vi "Acquisition Done.vi"(8 "error in (no error)":errorcluster, 11 "Picam in":refnum<class "Picam.lvclass">) -> (0 "error out":errorcluster, 2 "Done":bool, 3 "Picam out":refnum<class "Picam.lvclass">)   [LabVIEW 2019, in "Picam.lvclass"]
uses:
  Picam.lvclass
  Picam.lvclass/Picam.ctl
  picam32_LabView_SDK/PICam_lib/PICam.lvlib
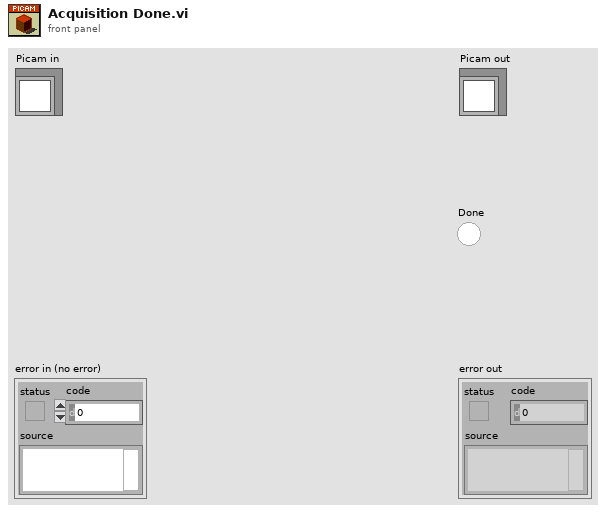
[diagram p1: front panel]
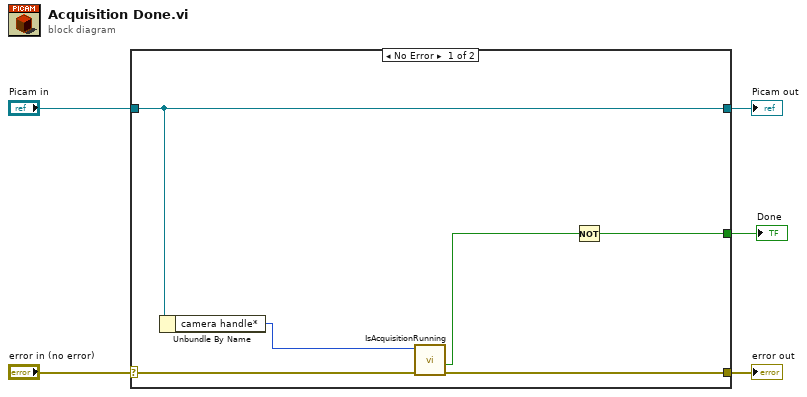
[diagram p0: block diagram]
diagram:
  n1 = case shown="No Error" "error in (no error)" {
    selector: "error in (no error)" -> [w11 w13]
    tunnel: [w10 w13] -> w4
    tunnel: [w9 w12] -> w2
    tunnel: "Picam in" -> [w9 w12]
    tunnel: [w6 _] -> w1
    frame No Error {
      n2 = Unbundle By Name(w9) -> ("camera handle*"=w8:u64)
      n3 = call "IsAcquisitionRunning.vi"("error in"=w11, "camera handle in"=w8) -> ("error out"=w10:errorcluster, "IsAcquisitionRunning"=w7:bool)  [unwired: 7 in, 1 out]
      n4 = Not(x=w7) -> (.not. x?=w6:bool)
    }
    frame Error {
    }
  }
  "error out" <- w4
  "Picam out" <- w2
  "Done" <- w1
